vi "GenerateListOfSuccessSpecsOrPreviewOrder.vi"(8 "error in (no error)":errorcluster, 9 "Generated file":T1, 11 "SolutionBuilder in":refnum<class "SolutionBuilder.lvclass">) -> (0 "error out":errorcluster, 1 "Builds":string[](array[string]), 3 "SolutionBuilder out":refnum<class "SolutionBuilder.lvclass">)   [LabVIEW 2019, in "SolutionBuilder.lvlib" / "SolutionBuilder.lvclass"]
uses:
  SolutionBuilder.lvclass
  BuildManager/GeneratedFile.ctl
  ProjectItem/ProjectItem.lvclass
  BuildManager/BuildManager.lvclass
  BuildManager/BuildProjectInfo.ctl
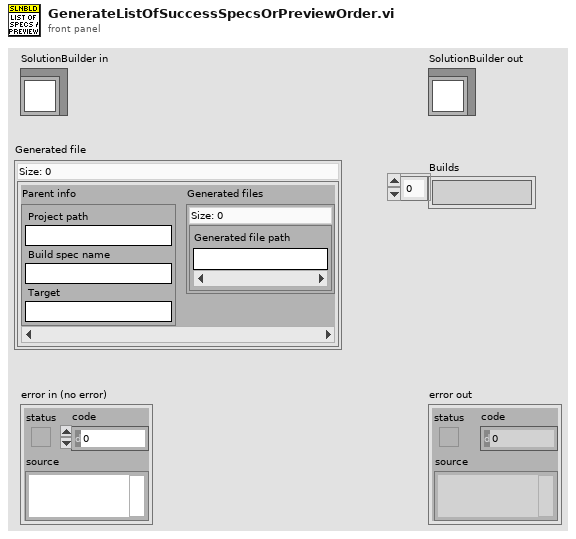
[diagram p1: front panel]
types:
  T1 = typedef "SolutionBuilder.lvlib/BuildManager.lvclass/GeneratedFile.ctl" = map{T2, set{string}}
  T2 = typedef "SolutionBuilder.lvlib/BuildManager.lvclass/BuildProjectInfo.ctl" = cluster{"Project path":string, "Build spec name":string, "Target":string}
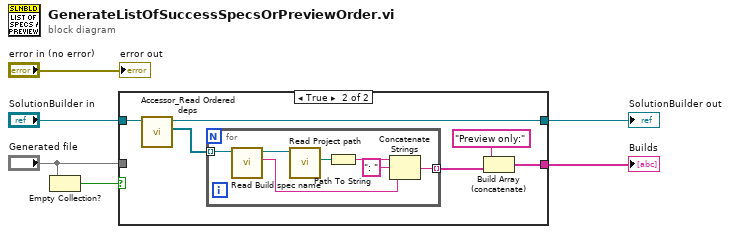
[diagram p0: block diagram]
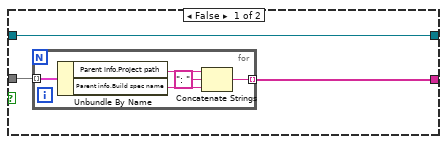
[diagram p2: hidden frame]
diagram:
  n1 = Empty Collection?(1:"Generated file") -> (0:w4:bool)
  n2 = case shown="True" w4 {
    tunnel: "Generated file" -> [w9 _]
    tunnel: [w8 w18] -> w3
    tunnel: "SolutionBuilder in" -> [w8 w19]
    tunnel: [w7 w16] -> w1
    frame False {
      n3 = for {
        tunnel: w9 -> [w14] mode=indexing
        tunnel: [w10] -> w7 mode=indexing
        n4 = Unbundle By Name(w14) -> ("Parent info.Project path"=w12:string, "Parent info.Build spec name"=w11:string)
        n5 = Concatenate Strings(w12, ": " ("string"), w11) -> (w10:string)
      }
    }
    frame True {
      n6 = call "Accessor_Read Ordered deps.vi"("SolutionBuilder in"=w19) -> ("Ordered deps"=w20:refnum<class "ProjectItem.lvclass">[], "SolutionBuilder out"=w18:refnum<class "SolutionBuilder.lvclass">)  [unwired: 8 in, 1 out]
      n7 = for {
        tunnel: w20 -> [w27] mode=indexing
        tunnel: [w24] -> w17 mode=indexing
        n8 = call "Read Build spec name.vi"("ProjectItem in"=w27) -> ("Build spec name"=w25:string, "ProjectItem out"=w23:refnum<class "ProjectItem.lvclass">)  [unwired: 9 in]
        n9 = call "Read Project path.vi"("ProjectItem in"=w23) -> ("Project path"=w22:path)  [unwired: 9 in, 1 out]
        n10 = Path To String(path=w22) -> (string=w21:string)
        n11 = Concatenate Strings(w21, ": " ("string"), w25) -> (w24:string)
      }
      n12 = Build Array (concatenate)("Preview only:" ("string"), w17) -> (w16:string[])
    }
  }
  "SolutionBuilder out" <- w3
  "Builds" <- w1
  "error out" <- "error in (no error)"
